vi "Died.vi"(8 "error in (no error)":errorcluster, 11 "JQMHModule in":refnum<class "RQMHModule.lvclass">) -> (0 "error out":errorcluster, 3 "JQMHModule out":refnum<class "RQMHModule.lvclass">)   [LabVIEW 2024, in "RQMHModule.lvclass"]
uses:
  RQMHModule.lvclass
  Shared/Died.ctl
  RQMHModule.lvclass/RQMHModule.ctl
  Shared/JQMHShared.lvlib
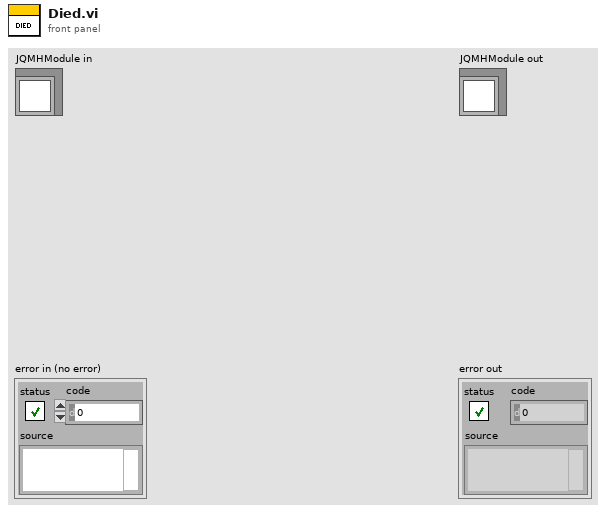
[diagram p1: front panel]
types:
  T1 = typedef "JQMHShared.lvlib/Died.ctl" = bool
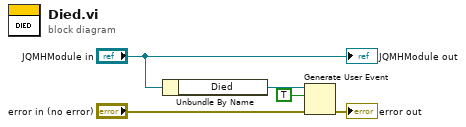
[diagram p0: block diagram]
diagram:
  n1 = Unbundle By Name("JQMHModule in") -> ("Died"=w4:refnum<user-event>)
  n2 = Generate User Event(user event=w4, event data cluster=T1 TRUE ("event data"), error in="error in (no error)") -> (error out=→"error out":errorcluster)  [unwired: 1 in, 1 out]
  "JQMHModule out" <- "JQMHModule in"
